vi "Set Receipt.vi"(8 "error in (no error)":errorcluster, 9 "CC":string[](array[string]), 10 "TO":string[](array[string]), 11 "Mail in":refnum<class "Mail.lvclass">) -> (0 "error out":errorcluster, 3 "Mail out":refnum<class "Mail.lvclass">)   [LabVIEW 2023, in "HardwareAbstractionLayer_LVOOP.lvlib" / "Mail.lvclass"]
uses:
  Mail.lvclass
  Mail.lvclass/Mail.ctl
  <vilib>/smtpClient/LabVIEWSMTPClient.lvlib
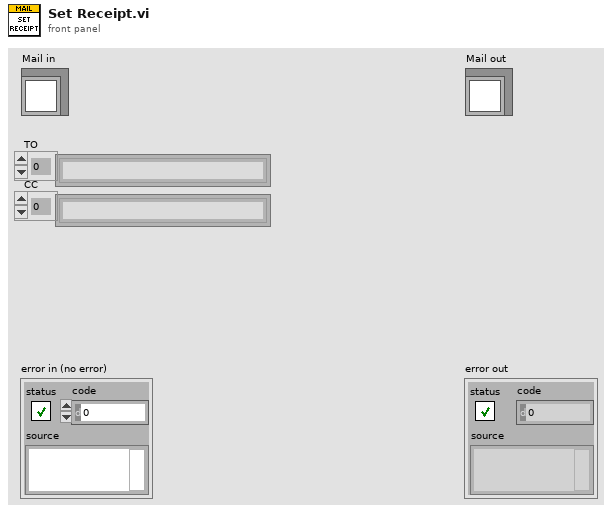
[diagram p1: front panel]
types:
  T1 = typedef "LabVIEWSMTPClient.lvlib/SmtpClientHandle.ctl" = refnum<k1>
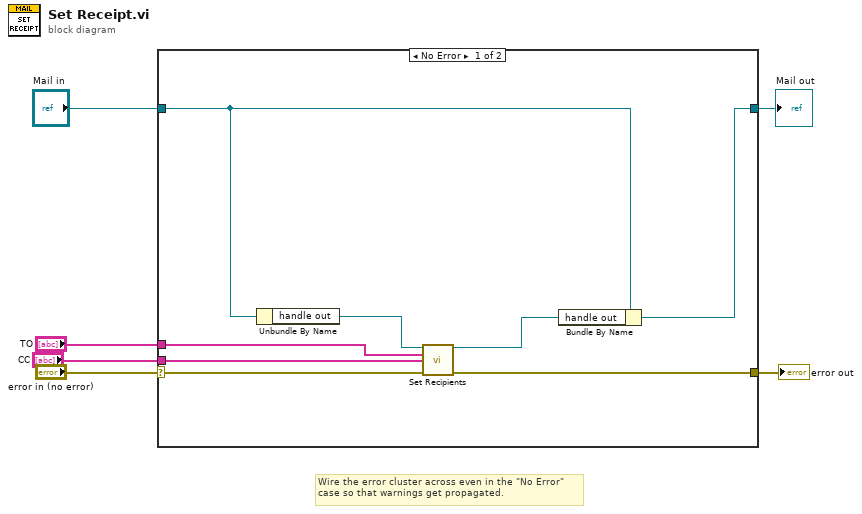
[diagram p0: block diagram]
diagram:
  # "Wire the error cluster across even in the \"No Error\"\ncase so that warnings get propagated."
  n1 = case shown="No Error" "error in (no error)" {
    selector: "error in (no error)" -> [w11 w16]
    tunnel: [w10 w16] -> w5
    tunnel: [w8 w15] -> w3
    tunnel: "Mail in" -> [w9 w15]
    tunnel: "TO" -> [w13 _]
    tunnel: "CC" -> [w12 _]
    frame No Error {
      n2 = Unbundle By Name(w9) -> ("handle out"=w14:T1)
      n3 = call <vilib>:"Set Recipients.vi"("handle in"=w14, "to"=w13, "cc"=w12, "error in (no error)"=w11) -> ("handle out"=w7:T1, "error out"=w10:errorcluster)  [unwired: 10 in]
      n4 = Bundle By Name(cluster=w9, "handle out"=w7) -> (w8:refnum<class "Mail.lvclass">)
    }
    frame Error {
    }
  }
  "error out" <- w5
  "Mail out" <- w3
